vi "rs3 open multiple sensor.vi"(0 "sensor in":u64, 5 "stream profile array":u64[](array[numeric]), 9 "Count of Streams":i32, 11 "error in (no error)":errorcluster) -> (4 "sensor out":u64, 10 "error":u64, 15 "error out":errorcluster)   [LabVIEW 2023]
doc: "This is where you CONFIGURE your SENSOR to stream some specific streams, by inputting array of the PROFILES (handles) that you want to stream \n\nINPUT:\nSensor in The sensor you want to stream from\nCount The number of streams you want the sensor to stream\nstream profile array The array containing the PROFILE handles that you want to stream"
panel:
  # "RS3 Open Multiple Sensor"
  # "(C) 2017 Intel Corp.,  AGJ"
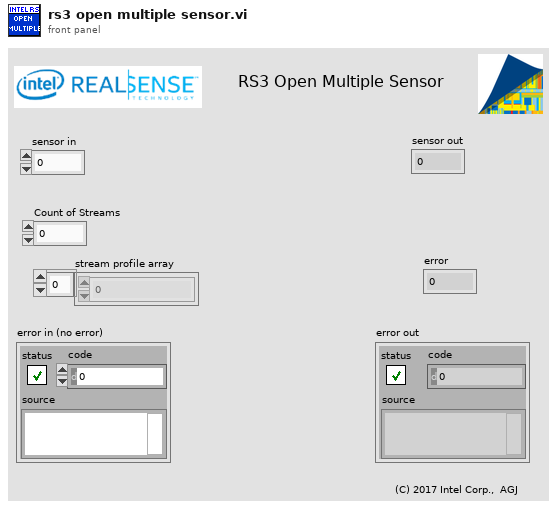
[diagram p1: front panel]
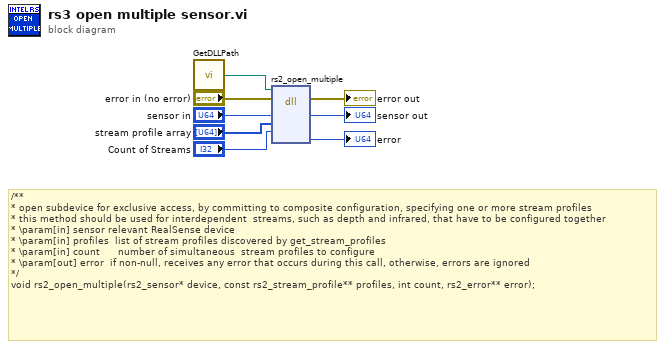
[diagram p0: block diagram]
diagram:
  # "/**\n* open subdevice for exclusive access, by committing to composite configuration, specifying one or more stream profiles\n* this method should be used for interdependent  streams, such as depth and infrared, that have to be configured together\n* \\param[in] sensor relevant RealSense device\n* \\param[in] profiles  list of stream profiles discovered by get_stream_profiles\n* \\param[in] count      number of simultaneous  stream profiles to configure\n* \\param[out] error  if non-null, receives any error that occurs during this call, otherwise, errors are ignored\n*/\nvoid rs2_open_multiple(rs2_sensor* device, const rs2_stream_profile** profiles, int count, rs2_error** error);"
  n1 = call "GetDLLPath.vi"() -> ("DLL Path"=w1:path)
  n2 = dll-call lib="C:/STEAMSyndicate/RealSenseWrappers/VI Wrappers (add ons) Public/RealSense/realsense2.dll" fn="rs2_open_multiple"(path in=w1, error in="error in (no error)", "sensor"="sensor in", "stream profile"="stream profile array", "count"="Count of Streams") -> (error out=→"error out":errorcluster, "sensor"=→"sensor out":u64, "error"=→"error":u64)  [unwired: 5 in, 1 out]
